vi "Temperature from File.vi"(0 "File Name:":path) -> (1 "File Path":path, 2 "Temperature set points":dbl[](graph))   [LabVIEW 2025]
doc: "This simple example reads the ASCII data files that were written with the Write Temperature to File VI. After the data string is read in, the data values are converted to numeric values and displayed on a graph. The file utility VIs are used to do all the file operations.\nAuthor: Scott Hannahs <sth@magnet.fsu.edu>\n\nThis software is licensed for use under the “MIT License\"\nCopyright (c) 2025 Scott Hannahs, sth@sth@magnet.sthnet.net\n\nPermission is hereby granted, free of charge, to any person obtaining a copy of this software and associated documentation files (the \"Software\"), to deal in the Software without restriction, including without limitation the rights to use, copy, modify, merge, publish, distribute, sublicense, and/or sell copies of the Software, and to permit persons to whom the Software is furnished to do so, subject to the following conditions: The above copyright notice and this permission notice shall be included in all copies or substantial portions of the Software.\n\nTHE SOFTWARE IS PROVIDED \"AS IS\", WITHOUT WARRANTY OF ANY KIND, EXPRESS OR IMPLIED, INCLUDING BUT NOT LIMITED TO THE WARRANTIES OF MERCHANTABILITY, FITNESS FOR A PARTICULAR PURPOSE AND NONINFRINGEMENT. IN NO EVENT SHALL THE AUTHORS OR COPYRIGHT HOLDERS BE LIABLE FOR ANY CLAIM, DAMAGES OR OTHER LIABILITY, WHETHER IN AN ACTION OF CONTRACT, TORT OR OTHERWISE, ARISING FROM, OUT OF OR IN CONNECTION WITH THE SOFTWARE OR THE USE OR OTHER DEALINGS IN THE SOFTWARE."
panel:
  out "String Read from File":string
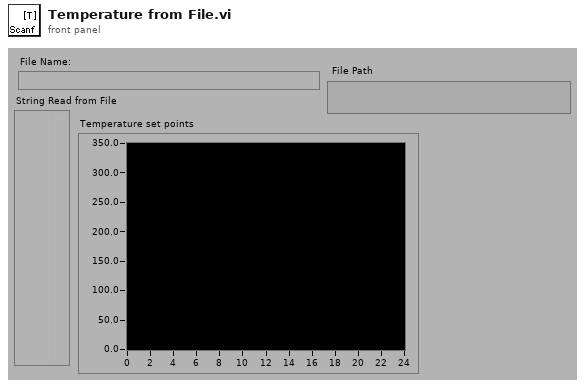
[diagram p1: front panel]
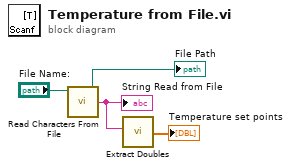
[diagram p0: block diagram]
diagram:
  n1 = call <vilib>:"Read Characters From File.vi"("file path (dialog if empty)"="File Name:") -> ("new file path (NotAPath if cancelled)"=→"File Path":path, "character string"=w3:string)  [unwired: 5 in, 2 out]
  "String Read from File" <- w3
  n2 = call "Extract Doubles.vi"("String"=w3) -> ("Data"=→"Temperature set points":dbl[])  [unwired: 5 in, 1 out]
